vi "Login.vi"(9 "error in (no error)":errorcluster) -> (1 "error out":errorcluster, 2 "Access Granted":bool)   [LabVIEW 2013]
doc: "This VI is the solution to Exercise 3-1 of the LabVIEW Basics II course.\n\nThis VI will accept a user name and password, and after the OK button is pressed, verify if the information is valid using the Verify Information subVI. The name and password controls are initialized to empty strings and the Key Focus attribute of the Login Name control is set to TRUE.\n\nYou will use this VI in Application Exercise.vi (Exercise 5-1) as your login screen."
uses:
  SourceCode/GlobalValue.vi
  <vilib>/Utility/config.llb/Read Key (String).vi
  <vilib>/Utility/config.llb/NI_LVConfig.lvlib
panel:
  out "User":string caption="值"
  out "ps":string caption="值"
  in  "Cancle":bool
  in  "Ok":bool
  in  "Password":string
  in  "Login Name":string
  # "用户登录"
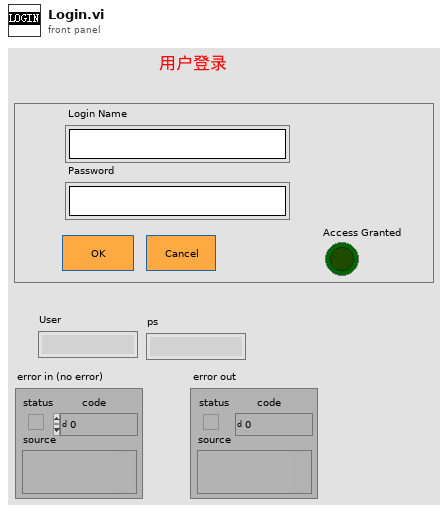
[diagram p1: front panel]
types:
  T1 = typedef "NI_LVConfig.lvlib/Config Data RefNum.ctl" = refnum<k1>
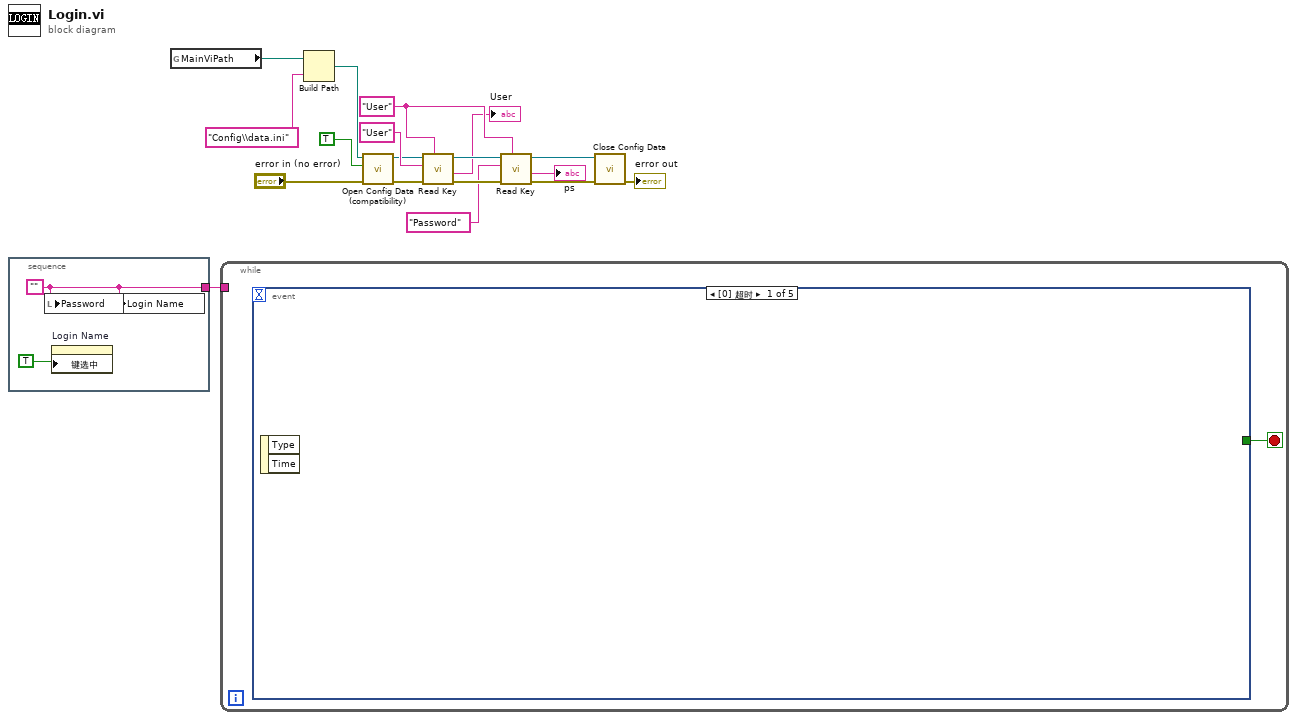
[diagram p0: block diagram]
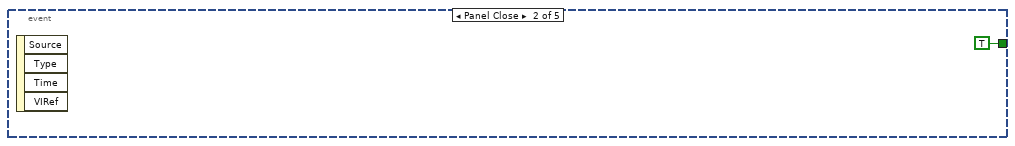
[diagram p2: hidden frame]
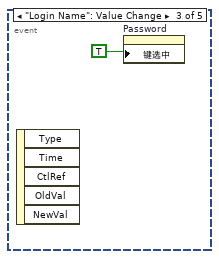
[diagram p3: hidden frame]
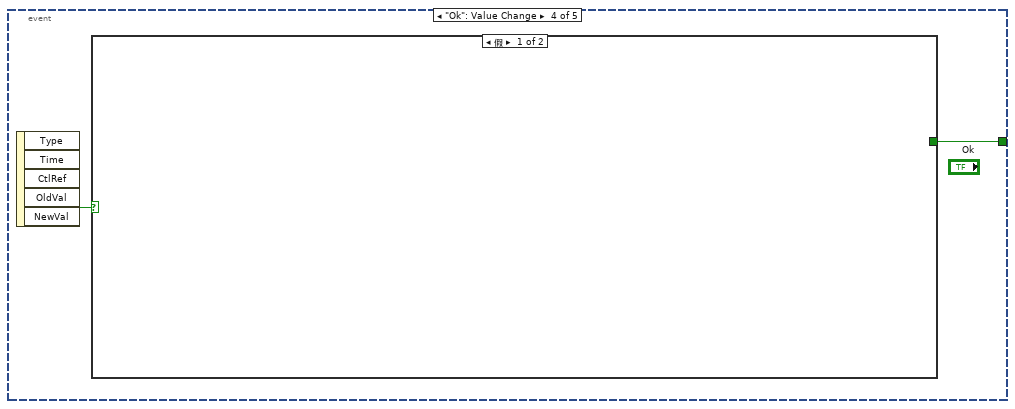
[diagram p4: hidden frame]
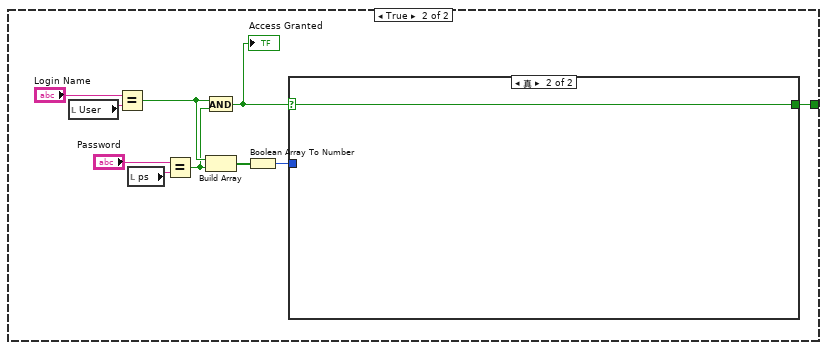
[diagram p5: hidden frame]
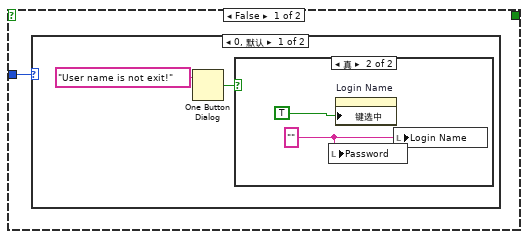
[diagram p6: hidden frame]
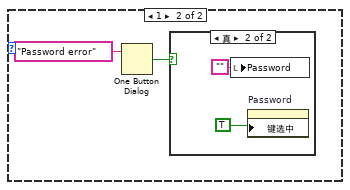
[diagram p8: hidden frame]
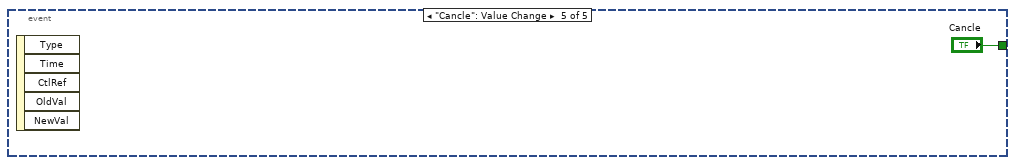
[diagram p10: hidden frame]
diagram:
  w11 = "User" ("ModelName")
  n1 = stacked-sequence {
    tunnel: [w19] -> w18
    frame #0 {
      w19 = ""
      n2 = local write "Password"(w19) -> ()
      n3 = property on="Login Name" class="Str"("键选中"=TRUE ("Key Focus")) -> ()  [unwired: 2 in, 2 out]
      n4 = local write "Login Name"(w19) -> ()
    }
  }
  n5 = global read "GlobalValue.vi" "MainViPath"() -> (w1:path)
  n6 = while {
    tunnel: w18 -> [_]
    stop <- w21 stop-if-true
    n7 = event shown="[0] 超时" {
      selector: _ -> [_ _ _ _ _]
      dyn-events: _ -> [_ _ _ _ _]
      timeout: _ -> [_ _ _ _ _]
      tunnel: [_ TRUE ("Cancle") _ w24 "Cancle"] -> w21
      event Timeout {
        n8 = event-data() -> ()  [unwired: 3 out]
      }
      event Panel Close {
        n9 = event-data() -> ()  [unwired: 5 out]
      }
      event "Login Name": Value Change {
        n10 = event-data() -> ()  [unwired: 6 out]
        n11 = property on="Password" class="Str"("键选中"=TRUE ("Key Focus")) -> ()  [unwired: 2 in, 2 out]
      }
      event "Ok": Value Change {
        n12 = event-data() -> ("NewVal"=w25:bool)  [unwired: 5 out]
        n13 = case shown="假" w25 {
          tunnel: [_ w35] -> w24
          frame False {
          }
          frame True {
            n14 = local read "User"() -> (w31:string)
            n15 = Equal?(x="Login Name", y=w31) -> (x = y?=w29:bool)
            n16 = local read "ps"() -> (w32:string)
            n17 = Equal?(x="Password", y=w32) -> (x = y?=w28:bool)
            n18 = And(x=w29, y=w28) -> (x .and. y?=w30:bool)
            "Access Granted" <- w30
            n19 = Build Array(w29, w28) -> (w27:bool[])
            n20 = Boolean Array To Number(Boolean array=w27) -> (number=w26:u32)
            n21 = case shown="真" w30 {
              selector: w30 -> [_ w45]
              tunnel: [_ w45] -> w35
              tunnel: w26 -> [w36 _]
              frame False {
                n22 = case shown="0, 默认" w36 {
                  frame 0, Default {
                    n23 = One Button Dialog(message="User name is not exit!" ("消息")) -> (true=w37:bool)  [unwired: 1 out]
                    n24 = case shown="真" w37 {
                      frame False {
                      }
                      frame True {
                        w39 = "" ("Login Name")
                        n25 = local write "Password"(w39) -> ()
                        n26 = property on="Login Name" class="Str"("键选中"=TRUE ("Key Focus")) -> ()  [unwired: 2 in, 2 out]
                        n27 = local write "Login Name"(w39) -> ()
                      }
                    }
                  }
                  frame 1 {
                    n28 = One Button Dialog(message="Password error" ("消息")) -> (true=w41:bool)  [unwired: 1 out]
                    n29 = case shown="真" w41 {
                      frame False {
                      }
                      frame True {
                        n30 = local write "Password"("") -> ()
                        n31 = property on="Password" class="Str"("键选中"=TRUE ("Key Focus")) -> ()  [unwired: 2 in, 2 out]
                      }
                    }
                  }
                }
              }
              frame True {
              }
            }
          }
        }
      }
      event "Cancle": Value Change {
        n32 = event-data() -> ()  [unwired: 6 out]
      }
    }
  }
  n33 = Build Path(base path=w1, name or relative path="Config\\data.ini" ("名称或相对路径")) -> (appended path=w15:path)
  n34 = call <vilib>:"Open Config Data (compatibility).vi"("error in (no error)"="error in (no error)", "create file if necessary (T)"=TRUE, "configuration file path"=w15) -> ("error out"=w7:errorcluster, "refnum"=w9:T1)  [unwired: 6 in, 1 out]
  n35 = call-poly <vilib>:"Read Key.vi"("section"=w11, "error in (no error)"=w7, "key"="User", "refnum"=w9) -> ("error out"=w12:errorcluster, "value"=→"User":string, "refnum out"=w13:T1)  [unwired: 2 in, 3 out]
  n36 = call-poly <vilib>:"Read Key.vi"("section"=w11, "error in (no error)"=w12, "key"="Password", "refnum"=w13) -> ("error out"=w2:errorcluster, "value"=→"ps":string, "refnum out"=w8:T1)  [unwired: 2 in, 3 out]
  n37 = call <vilib>:"Close Config Data.vi"("error in (no error)"=w2, "refnum"=w8) -> ("error out"=→"error out":errorcluster)  [unwired: 1 in, 8 out]
